vi "UTS - Calculate Message Timeout.vi"(9 "Result Parsing Timeout":i32, 10 "Message Timeout":i32, 11 "Module Timeout":i32) -> (3 "Calculated Timeout":i32)   [LabVIEW 2017]
uses:
  SSH.lvlib
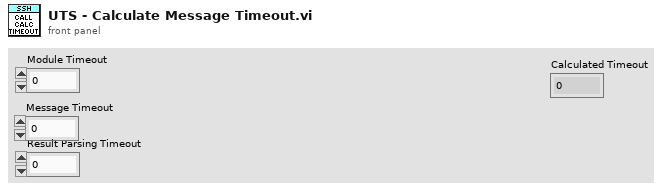
[diagram p1: front panel]
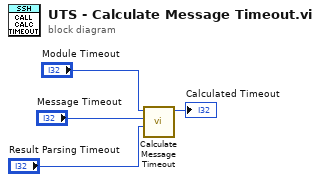
[diagram p0: block diagram]
diagram:
  n1 = call "Calculate Message Timeout.vi"("Result Parsing Timeout"="Result Parsing Timeout", "Message Timeout"="Message Timeout", "Module Timeout"="Module Timeout") -> ("Calculated Timeout"=→"Calculated Timeout":i32)  [unwired: 8 in]
